vi "MB_Master Simple Serial.vi"() -> ()   [LabVIEW 2012]
doc: "This VI demonstrates how to open a Modbus serial session and poll a single input register.\n\nBefore running, set the approptiate communication parameters and a valid input register address \nfrom your slave device."
uses:
  MB_Master_Serial/MB_Master_Serial.lvclass
  MB Master.lvlib
panel:
  out "error out":errorcluster
  in  "Poll Period (ms)":u32=1000
  out "Input Register Value":u16
  in  "stop":bool
  in  "Input Register Address":u16
  in  "Mode (RTU)":enum16{"RTU", "ASCII"}(ring)
  in  "Slave ID":u8=1
  in  "Serial Config":T1={"baud rate (bps)"=19200, "stop bits"=20, "parity"=0, "flow control"=0, "timeout"=1000, "retries"=1} {"stop bits" items=["1.0"=10, "1.5"=15, "2.0"=20]; "flow control" items=["None", "XON/XOFF", "RTS/CTS", "XON/XOFF & RTS/CTS", "DTR/DSR", "XON/XOFF & DTR/DSR"]; "parity" items=["None", "Odd", "Even", "Mark", "Space"]}
  in  "VISA Resource":refnum<visa-resource-name>
  # "This VI demonstrates how to open a Modbus serial session and poll a single input register.\n\nBefore running, set the approptiate communication parameters and a valid input register address \nfrom your slave device."
  # "Communication Parameters"
  # "Discrete Input Polling"
  # "Abort / Error"
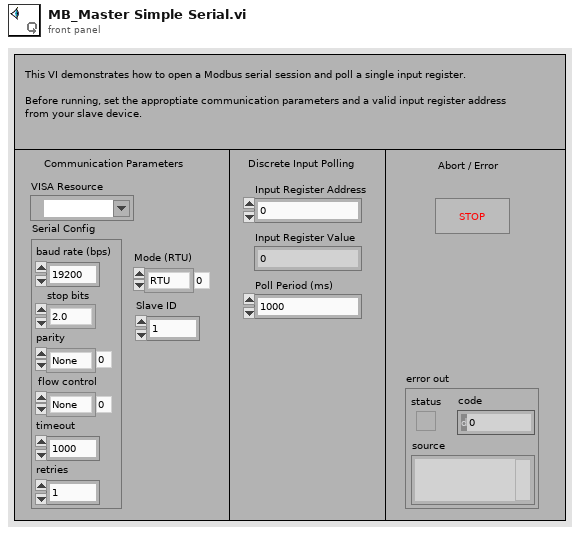
[diagram p1: front panel]
types:
  T1 = cluster{"baud rate (bps)":u32, "stop bits":u16, "parity":u16, "flow control":u16, "timeout":u32, "retries":i32}
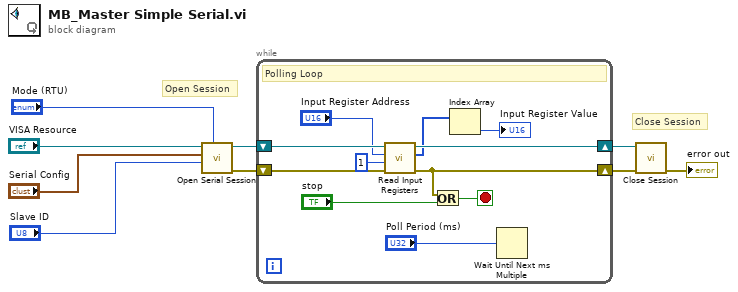
[diagram p0: block diagram]
diagram:
  # "Close Session"
  # "Open Session"
  n1 = call "Open Serial Session.vi"("Mode (RTU)"="Mode (RTU)", "Slave ID"="Slave ID", "Serial Config"="Serial Config", "VISA Resource"="VISA Resource") -> ("Error out"=w4:errorcluster, "MB_Serial session"=w5:refnum<class "MB_Master_Serial.lvclass">)  [unwired: 6 in]
  n2 = while {
    shift-right: [w16] -> w3
    shift-left: w5 -> [w20]
    shift-right: [w14] -> w2
    shift-left: w4 -> [w19]
    stop <- w13 stop-if-true
    # "Polling Loop"
    n3 = call "Read Input Registers.vi"("error in (no error)"=w19, "quantity"=u16 1, "starting address"="Input Register Address", "MB session in"=w20) -> ("error out"=w14:errorcluster, "Registers"=w12:u16[], "MB session out"=w16:refnum<class "MB_Master_Serial.lvclass">)  [unwired: 5 in]
    n4 = Or(x=w14, y="stop") -> (x .or. y?=w13:bool)
    n5 = Index Array(array=w12) -> (element=→"Input Register Value":u16)  [unwired: 1 in]
    n6 = Wait Until Next ms Multiple(millisecond multiple="Poll Period (ms)") -> ()  [unwired: 1 out]
  }
  n7 = call-dynamic "Close Session.vi"("error in (no error)"=w2, "MB_Serial session"=w3) -> ("error out"=→"error out":errorcluster)  [unwired: 9 in]
